vi "日志存储 (子VI).vi"(11 "data in":T1) -> ()   [LabVIEW 2016, in "超标留样集成.lvlib" / "德润DR803M超标留样.lvlib"]
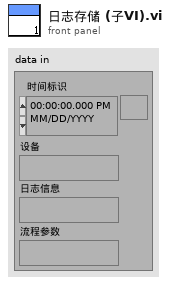
[diagram p1: front panel]
types:
  T1 = cluster{"时间标识":timestamp, "设备":string, "日志信息":string, "流程参数":string}
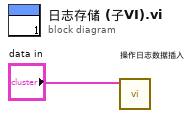
[diagram p0: block diagram]
diagram:
  n1 = call "操作日志数据插入.vi"("data"="data in") -> ()  [unwired: 9 in, 1 out]
